vi "feedback_with_message_channel.vi"() -> ()   [LabVIEW 2021]
uses:
  <extravilib>/ChannelInstances/Messenger-dbl/Write With Abort.vi
  <extravilib>/ChannelInstances/Messenger-dbl/Read With Abort.vi
  <extravilib>/ChannelInstances/Messenger-dbl/Instantiate.vi
  <extravilib>/ChannelInstances/Messenger-dbl/Endpoint.vi
  <extravilib>/ChannelInstances/Messenger-dbl.lvlib
panel:
  out "Waveform Chart":dbl(graph)
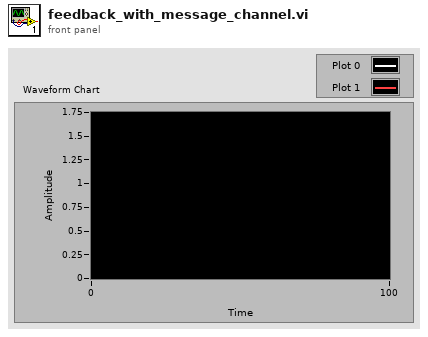
[diagram p1: front panel]
types:
  T1 = typedef "Messenger-dbl.lvlib/))Channel.ctl" = refnum<queue>
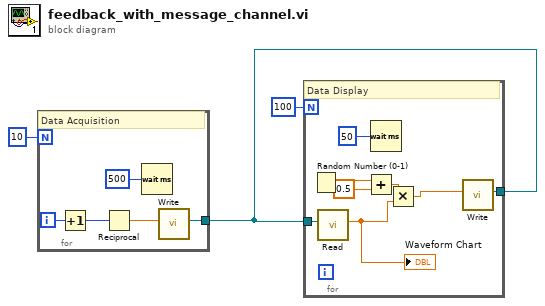
[diagram p0: block diagram]
diagram:
  n1 = for {
    N: 10 -> [_]
    tunnel: [w5] -> w1
    i -> [w7]
    # "Data Acquisition"
    n2 = Increment(x=w7) -> (x+1=w4:i32)
    n3 = Reciprocal(x=w4) -> (1/x=w6:dbl)
    n4 = Wait (ms)(milliseconds to wait=u32 500) -> ()  [unwired: 1 out]
    n5 = call <extravilib>:"Write.vi"("element"=w6) -> ("channel"=w5:T1)  [unwired: 8 in, 2 out]
  }
  n6 = for {
    N: 100 -> [_]
    tunnel: w1 -> [w15]
    tunnel: w1 -> [w14]
    # "Data Display"
    n7 = Random Number (0-1)() -> (number: 0 to 1=w13:dbl)
    n8 = call <extravilib>:"Read.vi"("channel"=w15) -> ("element"=w10:dbl)  [unwired: 8 in, 2 out]
    "Waveform Chart" <- w10
    n9 = Add(x=w13, y=0.5) -> (x+y=w11:dbl)
    n10 = Wait (ms)(milliseconds to wait=u32 50) -> ()  [unwired: 1 out]
    n11 = Multiply(x=w11, y=w10) -> (x*y=w9:dbl)
    n12 = call <extravilib>:"Write.vi"("element"=w9) -> ("channel"=w14:T1)  [unwired: 8 in, 2 out]
  }
